vi "FPGAmain_5782_Dual_PID_v3.vi"() -> ()   [LabVIEW 2013]
uses:
  FPGA/DataMode.ctl
  FPGA/Input_5782/5782_states.ctl
  <vilib>/Platform/TimedLoop/XDataNode/timing_clust.ctl
  <vilib>/Platform/TimedLoop/XDataNode/nitl_modes.ctl
  <vilib>/Platform/TimedLoop/XDataNode/wakeup.ctl
  <vilib>/rvi/Emulation/niFpgaSctlEmulationGetInTimedLoop.vi
  <vilib>/rvi/Emulation/niFpgaEmulationReportErrorSimple.vi
  <vilib>/rvi/Emulation/niFpgaGetClockAttributes.vi
  <vilib>/rvi/eio/common/nirviEmuTemplateMethod_errors.vi
  <vilib>/rvi/Emulation/niFpgaCriticalErrorInLSC.vi
  <vilib>/rvi/DataTransferAndStorage/Register/Emulation/niFpgaRegisterEmulationFpgaImpl.vi
  <instcachedir>/0/niFpgaRegisterEmulationFpgaImpl_DCF4BC0110594B98B44A971D60CEEC4D.lvgen/niFpgaRegisterEmulationFpgaImpl_DCF4BC0110594B98B44A971D60CEEC4D_011.vi
  <vilib>/rvi/DataTransferAndStorage/Container/Common/niFpgaContainerGetUniqueNameForEmu.vi
  <instcachedir>/0/niFpgaRegisterEmulationFpgaImpl_DCF4BC0110594B98B44A971D60CEEC4D.lvgen/niFpgaRegisterEmulationFpgaImpl_DCF4BC0110594B98B44A971D60CEEC4D_012.vi
  <instcachedir>/0/niFpgaRegisterEmulationFpgaImpl_DCF4BC0110594B98B44A971D60CEEC4D.lvgen/niFpgaRegisterEmulationFpgaImpl_DCF4BC0110594B98B44A971D60CEEC4D_003.vi
  <instcachedir>/0/niFpgaRegisterEmulationFpgaImpl_DCF4BC0110594B98B44A971D60CEEC4D.lvgen/niFpgaRegisterEmulationFpgaImpl_DCF4BC0110594B98B44A971D60CEEC4D_007.vi
  <instcachedir>/0/niFpgaRegisterEmulationFpgaImpl_DCF4BC0110594B98B44A971D60CEEC4D.lvgen/niFpgaRegisterEmulationFpgaImpl_DCF4BC0110594B98B44A971D60CEEC4D_008.vi
  <instcachedir>/0/niFpgaRegisterEmulationFpgaImpl_DCF4BC0110594B98B44A971D60CEEC4D.lvgen/niFpgaRegisterEmulationFpgaImpl_DCF4BC0110594B98B44A971D60CEEC4D_021.vi
  <instcachedir>/0/niFpgaRegisterEmulationFpgaImpl_DCF4BC0110594B98B44A971D60CEEC4D.lvgen/niFpgaRegisterEmulationFpgaImpl_DCF4BC0110594B98B44A971D60CEEC4D_020.vi
  <instcachedir>/0/niFpgaRegisterEmulationFpgaImpl_DCF4BC0110594B98B44A971D60CEEC4D.lvgen/niFpgaRegisterEmulationFpgaImpl_DCF4BC0110594B98B44A971D60CEEC4D_009.vi
  <vilib>/rvi/FIFO/Fifo_Resource/nirvififoEmulationReadFpgaImpl.vi
  <vilib>/rvi/interface/RandomDataEmulation/nirviRandomDataMultiElementFPGAFIFO.vi
  <instcachedir>/0/nirviRandomDataMultiElementFPGAFIFO_F2B80EDE0D7944A08478D8D26097D4DB.lvgen/nirviRandomDataMultiElementFPGAFIFO_F2B80EDE0D7944A08478D8D26097D4DB_005.vi
  <vilib>/rvi/interface/RandomDataEmulation/niFpgaRandomDataHandleErrors.vi
  <instcachedir>/0/niFpgaRegisterEmulationFpgaImpl_DCF4BC0110594B98B44A971D60CEEC4D.lvgen/niFpgaRegisterEmulationFpgaImpl_DCF4BC0110594B98B44A971D60CEEC4D_013.vi
  <vilib>/rvi/interface/RandomDataEmulation/nirviRandomDataFPGAFIFO.vi
  <vilib>/rvi/FIFO/Fifo_Resource/nirvififoEmulationWriteFpgaImpl.vi
  <vilib>/Platform/TimedLoop/XDataNode/XDataNode.xnode
  <vilib>/eio/EIONode/EIONode.xnode
  <vilib>/rvi/DataTransferAndStorage/Container/XNode/niFpgaContainer.xnode
  <vilib>/rvi/DataTransferAndStorage/Register/Emulation/niFpgaRegisterEmulation.vi
  <vilib>/rvi/FIFO/Fifo_Resource/nirvififoEmulationRead.vi
  <vilib>/rvi/interface/RandomDataEmulation/nirviRandomDataFpgaMultiElementTemplate.vi
  <vilib>/rvi/interface/RandomDataEmulation/nirviRandomDataFpgaReadWriteTemplate.vi
  <vilib>/rvi/FIFO/Fifo_Resource/nirvififoEmulationWrite.vi
  <vilib>/Platform/TimedLoop/XDataNode/XDNodeRunTimeDep.lvlib
panel:
  in  "IO Module\\AO Data Sync":bool=TRUE
  in  "IO Module\\SPI Write Data":u16
  out "IO Module\\SPI Read Data":u8
  in  "IO Module\\SPI Read":bool
  in  "IO Module\\SPI Write":bool
  in  "IO Module\\SPI Address":u16
  in  "IO Module\\SPI Device":u8
  out "IO Module\\SPI Idle":bool
  in  "AM phase":fxp<+,64,64>
  in  "delay phase":fxp<+,64,64>
  in  "User Command Commit":bool
  in  "User Command":u8
  out "User Command Idle":bool
  out "User Command Status":u8
  in  "User Data 0":u8
  in  "User Data 1":u8
  out "PLL Locked":bool
  out "User Error":bool
  out "Configured?":bool
  in  "Continuous":bool
  in  "5782 record length":u16=4000 caption="Samples Per Trigger" min=1 step=1
  in  "Trigger Acquisition":bool
  out "IO Module\\Trigger Input":bool
  in  "Downsample":fxp<+,8,8>=1.0
  in  "new coeffs":bool
  in  "FIR coeffs":fxp<+/-,18,18>[](array[numeric])
  in  "CIC Gain":fxp<+/-,32,1>=0.00390625 format="%#_32g"
  in  "Acquisition running":bool
  in  "Phase output":fxp<+,64,64>[](array[numeric])=[0.0, 0.0, 0.0, 0.0, 0.0, 0.0, 0.0, 0.0]
  in  "Simulated phase 5782":fxp<+,64,64>[](array[numeric])=[0.0, 0.0]
  in  "Mode":T1
  in  "Phase 5782":fxp<+,64,64>[](array[numeric])=[0.0, 0.0]
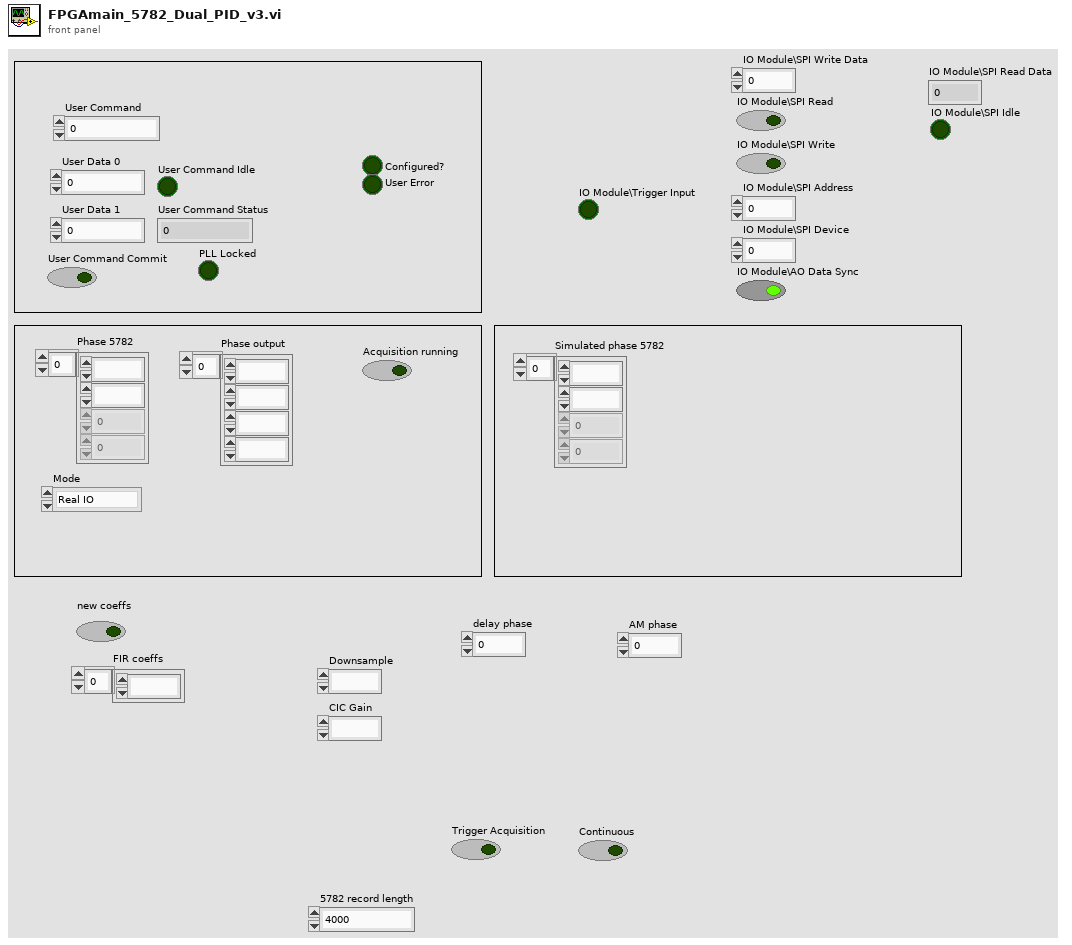
[diagram p1: front panel]
types:
  T1 = typedef "DataMode.ctl" = enum16{"Real IO", "Simulated"}
  T2 = typedef "5782_states.ctl" = enum8{"Wait for trigger", "Acquisition", "Send record length", "Quiet period"}
  T3 = typedef "XDNodeRunTimeDep.lvlib/timing_clust.ctl" = cluster{"Expected End [f-1]":u64, "Actual End [f-1]":u64, "Finished Late? [f-1]":bool, "Expected End [i-1]":u64, "Actual End [i-1]":u64, "Finished Late? [i-1]":bool, "Expected Start [i]":u64, "Actual Start [i]":u64, "Expected Start [f]":u64, "Actual Start [f]":u64, "Source Name":string, "Structure Name":string, "Period":i64, "Deadline":i64, "Offset":i64, "Start":i64, "Priority":i32, "Timeout":i32, "Mode":T4, "Wakeup Reason":T5, "Error":errorcluster, "Source Type":string, "Secondary Source Type":string, "Global End Time":u64, "Global Start Time":u64, "Frame Duration":u64, "Iteration Duration":u64, "Assigned CPU":i32, "I/O Scan Engine Mode":u32}
  T4 = typedef "XDNodeRunTimeDep.lvlib/nitl_modes.ctl" = enum32{"No Change", "Process missed periods, maintain original phase", "Discard missed periods, maintain original phase", "Process missed periods, ignore original phase", "Discard missed periods, ignore original phase"}
  T5 = typedef "XDNodeRunTimeDep.lvlib/wakeup.ctl" = enum32{"Normal", "Aborted", "Asynchronous wakeup", "Timing source error", "Timed loop error", "Timeout"}
  T6 = typedef "I16 array size 2.ctl" = i16[]
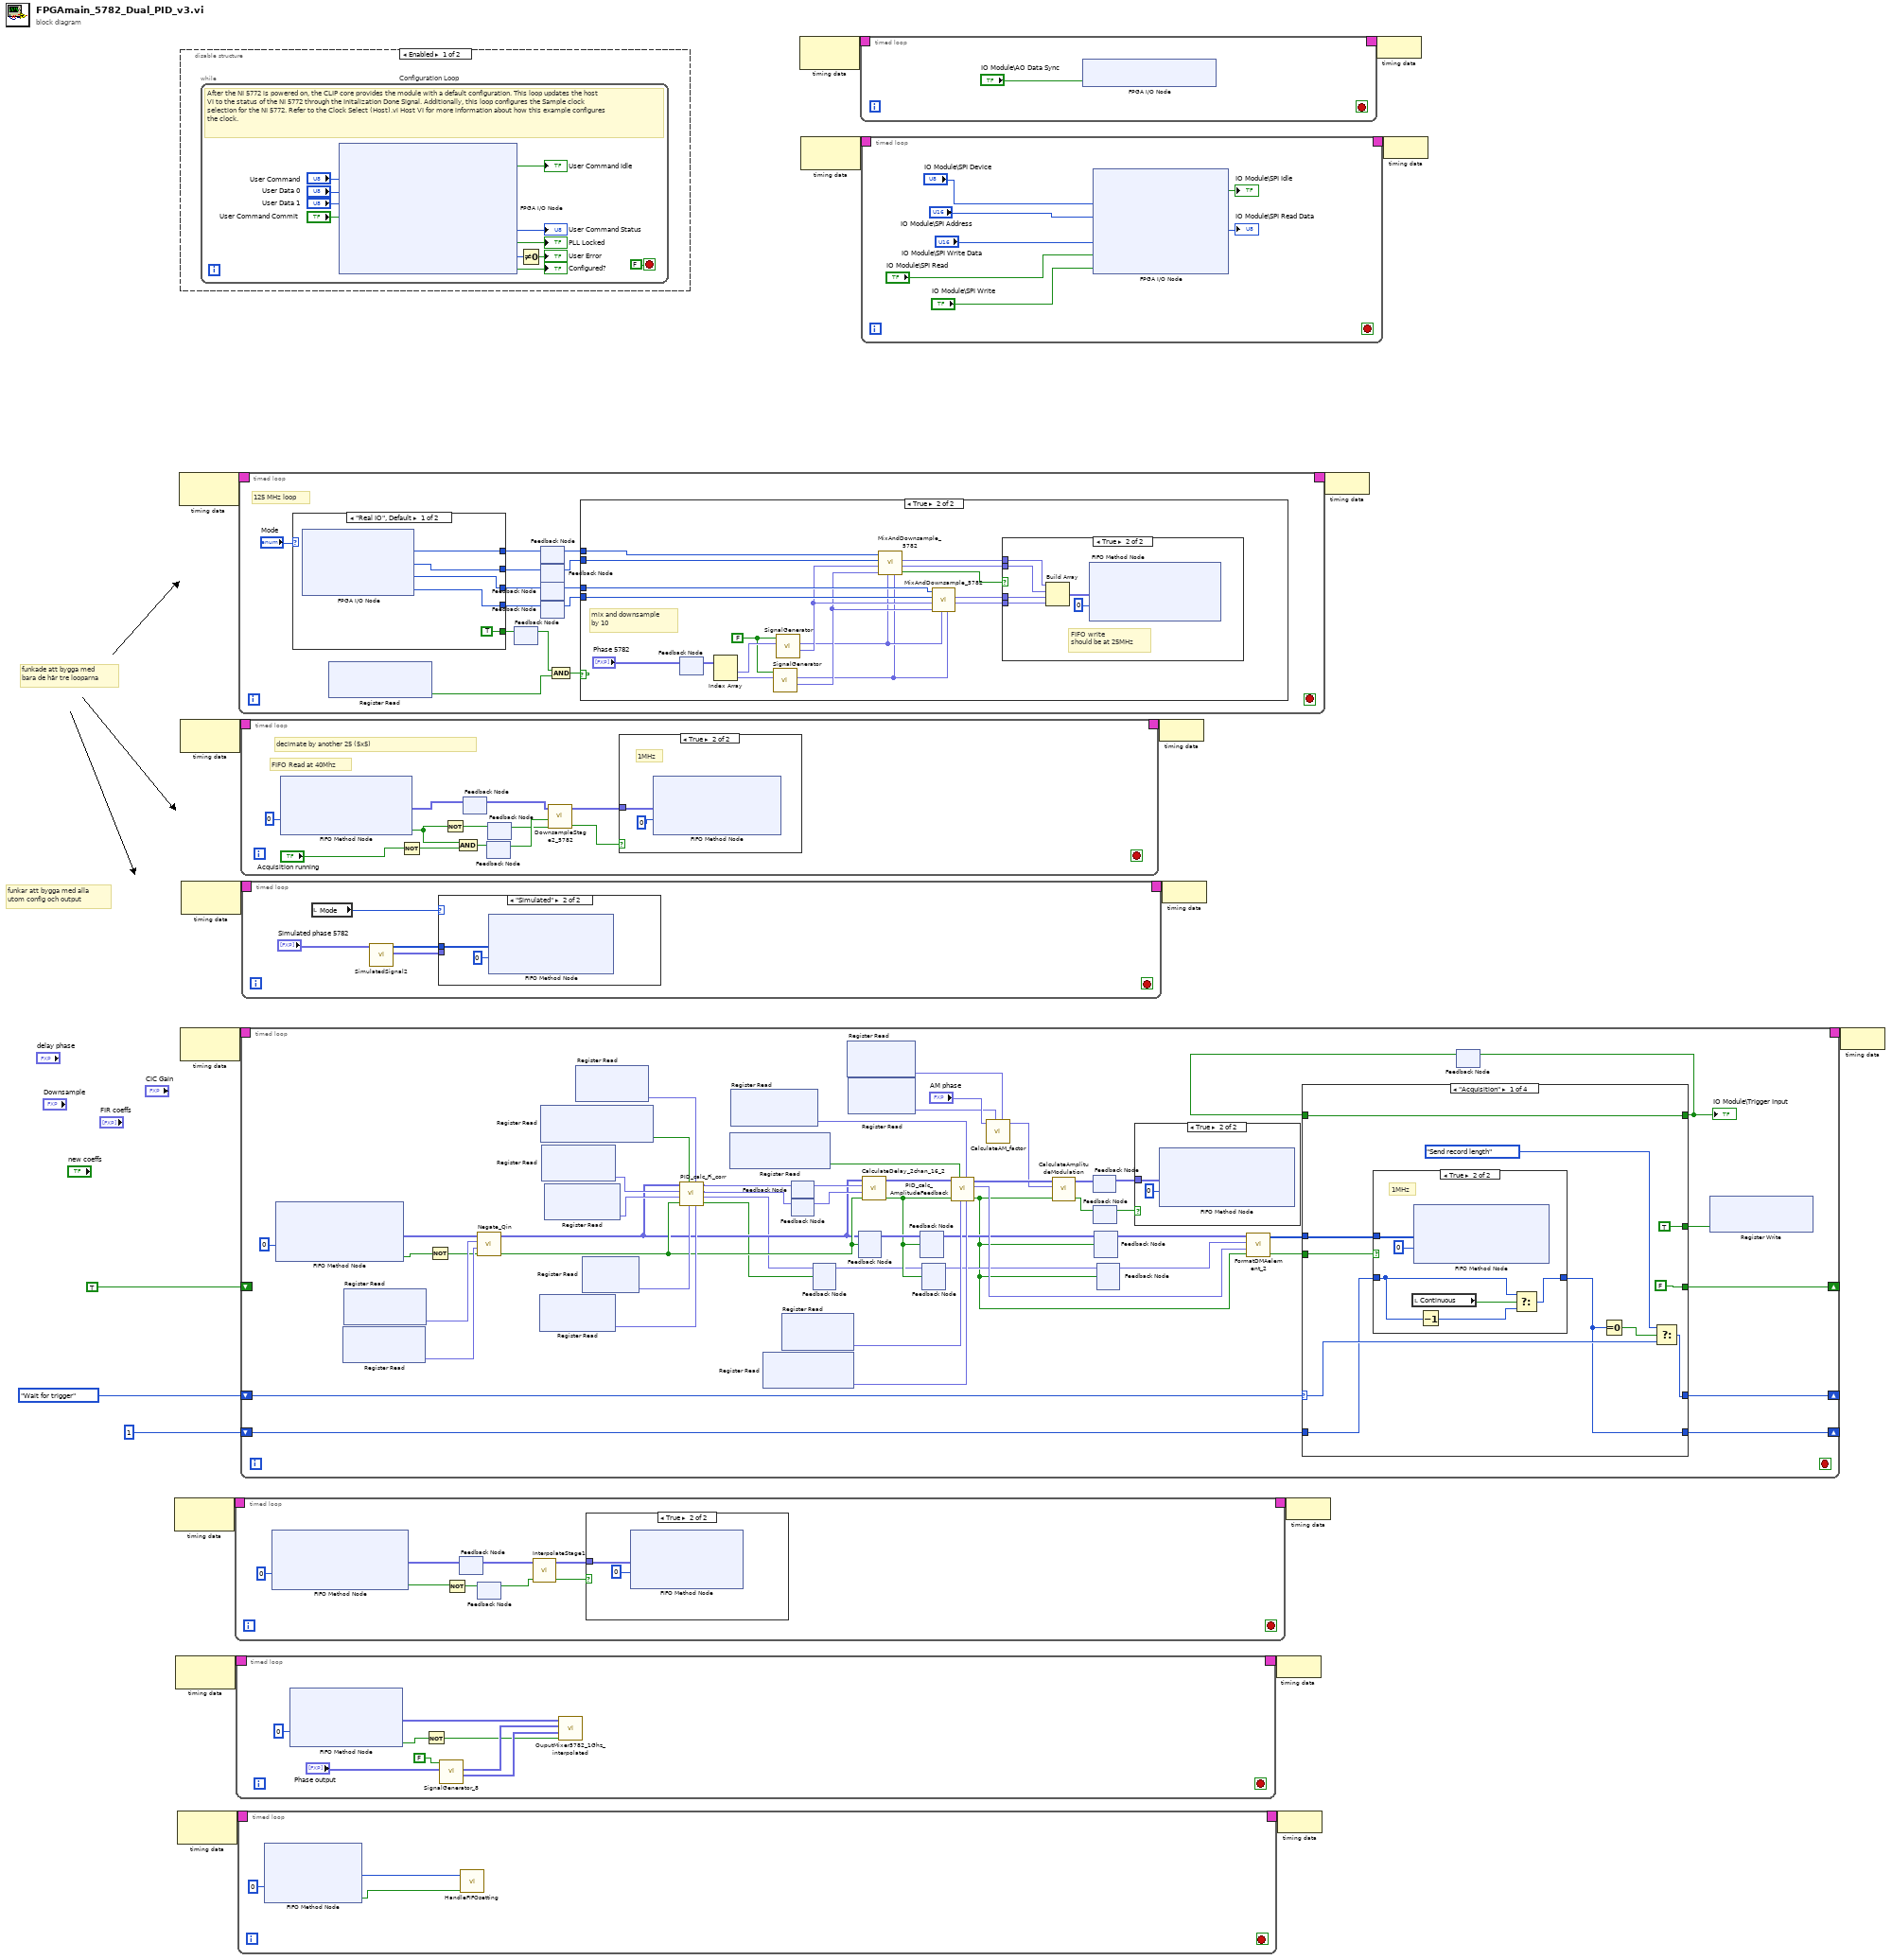
[diagram p0: block diagram]
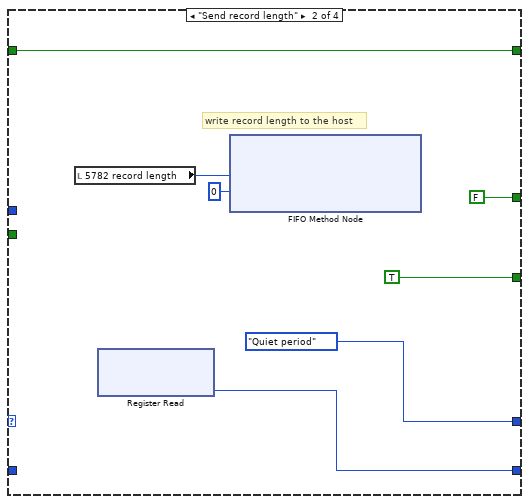
[diagram p5: hidden frame]
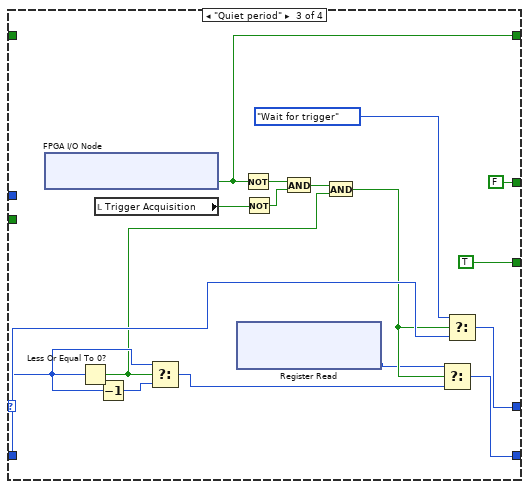
[diagram p6: hidden frame]
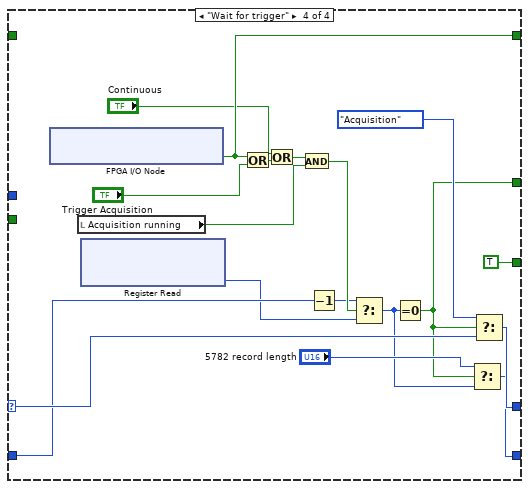
[diagram p7: hidden frame]
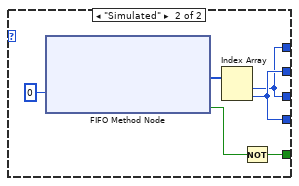
[diagram p11: hidden frame]
diagram:
  # "funkar att bygga med alla\nutom config och output"
  # "funkade att bygga med\nbara de här tre looparna"
  n1 = node-c288() -> (w2:T3)  [unwired: 1 in]
  n2 = node-c288() -> (w8:T3)  [unwired: 1 in]
  n3 = node-c288() -> (w10:T3)  [unwired: 1 in]
  n4 = node-c288() -> (w17:T3)  [unwired: 1 in]
  n5 = disable-structure shown="Enabled" {
    frame Enabled {
      n6 = while "Configuration Loop" {
        stop <- FALSE stop-if-true
        # "After the NI 5772 is powered on, the CLIP core provides the module with a default configuration. This loop updates the host VI to the status of the NI 5772 through the Initalization Done Signal. Additionally, this loop configures the Sample clock selection for the NI 5772. Refer to the Clock Select (Host).vi Host VI for more information about how this example configures the clock."
        n7 = xnode "FPGA I/O Node"("IO Module\\User Command"="User Command", "IO Module\\User Data 0"="User Data 0", "IO Module\\User Data 1"="User Data 1", "IO Module\\User Command Commit"="User Command Commit") -> ("IO Module\\User Command Idle"=→"User Command Idle":bool, "IO Module\\User Command Status"=→"User Command Status":u8, "IO Module\\PLL Locked"=→"PLL Locked":bool, "IO Module\\User Error"=w27:u8, "IO Module\\Initialization Done"=→"Configured?":bool)  [unwired: 9 in, 9 out]
        n8 = Not Equal To 0?(x=w27) -> (x != 0?=→"User Error":bool)
      }
    }
    frame Disabled {
    }
  }
  n9 = node-c288() -> (w21:T3)  [unwired: 1 in]
  n10 = node-c288() -> (w15:T3)  [unwired: 1 in]
  n11 = node-c288() -> (w19:T3)  [unwired: 1 in]
  n12 = timed-loop {
    timing: w2 -> [_]
    timing-out: [_] -> w1
    stop <- _ stop-if-true
    n13 = xnode ("FIFO Method Node")("Timeout"=0) -> ("Element"=w34:fxp<+/-,16,14>[], "Timed Out?"=w39:bool)  [unwired: 1 in, 1 out]
    n14 = Not(x=w39) -> (.not. x?=w36:bool)
    n15 = feedback #1() -> (w33:fxp<+/-,16,14>[])  [unwired: 1 in]
    n16 = feedback-in #1(w34) -> ()
    n17 = feedback #2() -> (w35:bool)  [unwired: 1 in]
    n18 = feedback-in #2(w36) -> ()
    n19 = call "InterpolateStage1.vi"("valid in"=w35, "Data in"=w33) -> ("valid out"=w38:bool, "Data out"=w37:fxp<+/-,16,14>[])  [unwired: 8 in]
    n20 = case shown="True" w38 {
      tunnel: w37 -> [_ w42]
      frame False {
      }
      frame True {
        n21 = xnode ("FIFO Method Node")("Element"=w42, "Timeout"=0) -> ()  [unwired: 1 in, 2 out]
      }
    }
  }
  n22 = timed-loop {
    timing: w8 -> [_]
    timing-out: [_] -> w7
    stop <- _ stop-if-true
    n23 = xnode ("FIFO Method Node")("Timeout"=0) -> ("Element"=w46:fxp<+/-,16,14>[], "Timed Out?"=w51:bool)  [unwired: 1 in, 1 out]
    n24 = Not(x=w51) -> (.not. x?=w45:bool)
    n25 = call "SignalGenerator_8.vi"("Phase"="Phase output", "reset"=FALSE) -> ("Sine out"=w47:fxp<+/-,16,0>[], "Cosine out"=w48:fxp<+/-,16,0>[])  [unwired: 8 in]
    n26 = call "OuputMixer5782_1Ghz_interpolated.vi"("input valid"=w45, "Sine in"=w47, "Cosine in"=w48, "Data"=w46) -> ()  [unwired: 7 in, 1 out]
  }
  n27 = timed-loop {
    timing: w10 -> [_]
    timing-out: [_] -> w9
    stop <- _ stop-if-true
    n28 = xnode ("FIFO Method Node")("Timeout"=0) -> ("Element"=w56:u64, "Timed Out?"=w55:bool)  [unwired: 1 in, 1 out]
    n29 = call "HandleFIFOsetting.vi"("timed out"=w55, "Value"=w56) -> ()  [unwired: 10 in]
  }
  n30 = timed-loop {
    timing: w17 -> [_]
    timing-out: [_] -> w16
    stop <- _ stop-if-true
    # "125 MHz loop"
    n31 = case shown="\"Real IO\", Default" "Mode" {
      tunnel: [w101 w104] -> w70
      tunnel: [w100 w105] -> w68
      tunnel: [w99 w104] -> w66
      tunnel: [w98 w105] -> w63
      tunnel: [TRUE w102] -> w62
      frame "Real IO", Default {
        n32 = xnode "FPGA I/O Node"() -> ("IO Module\\AI 0 N-1"=w101:i16, "IO Module\\AI 0 N"=w100:i16, "IO Module\\AI 1 N-1"=w99:i16, "IO Module\\AI 1 N"=w98:i16)  [unwired: 4 in, 4 out]
      }
      frame "Simulated" {
        n33 = xnode ("FIFO Method Node")("Timeout"=0) -> ("Element"=w106:i16[], "Timed Out?"=w103:bool)  [unwired: 1 in, 1 out]
        n34 = Index Array(array=w106) -> (element #1=w104:i16, element #2=w105:i16)  [unwired: 2 in]
        n35 = Not(x=w103) -> (.not. x?=w102:bool)
      }
    }
    n36 = xnode ("Register Read")() -> ("Data"=w60:bool)  [unwired: 1 in, 1 out]
    n37 = feedback #3() -> (w61:bool)  [unwired: 1 in]
    n38 = feedback-in #3(w62) -> ()
    n39 = feedback #4() -> (w69:i16)  [unwired: 1 in]
    n40 = feedback-in #4(w70) -> ()
    n41 = feedback #5() -> (w67:i16)  [unwired: 1 in]
    n42 = feedback-in #5(w68) -> ()
    n43 = feedback #6() -> (w65:i16)  [unwired: 1 in]
    n44 = feedback-in #6(w66) -> ()
    n45 = feedback #7() -> (w64:i16)  [unwired: 1 in]
    n46 = feedback-in #7(w63) -> ()
    n47 = And(x=w61, y=w60) -> (x .and. y?=w71:bool)
    n48 = case shown="True" w71 {
      tunnel: w69 -> [_ w80]
      tunnel: w67 -> [_ w79]
      tunnel: w65 -> [_ w78]
      tunnel: w64 -> [_ w77]
      frame False {
      }
      frame True {
        w81 = FALSE
        # "mix and downsample\nby 10"
        n49 = feedback #8() -> (w84:fxp<+,64,64>[])  [unwired: 1 in]
        n50 = feedback-in #8("Phase 5782") -> ()
        n51 = Index Array(array=w84) -> (element #1=w83:fxp<+,64,64>, element #2=w85:fxp<+,64,64>)  [unwired: 2 in]
        n52 = call "SignalGenerator.vi"("phase"=w85, "Reset"=w81) -> ("Cos"=w75:fxp<+/-,16,0>, "Sin"=w73:fxp<+/-,16,0>)  [unwired: 7 in, 1 out]
        n53 = call "SignalGenerator.vi"("phase"=w83, "Reset"=w81) -> ("Cos"=w76:fxp<+/-,16,0>, "Sin"=w74:fxp<+/-,16,0>)  [unwired: 7 in, 1 out]
        n54 = call "MixAndDownsample_5782.vi"("sin1"=w73, "sin0"=w74, "cos1"=w75, "cos0"=w76, "signal 1"=w79, "signal 0"=w80) -> ("data valid"=w88:bool, "Q out"=w89:fxp<+/-,16,14>, "I out"=w90:fxp<+/-,16,14>)  [unwired: 3 in]
        n55 = call "MixAndDownsample_5782.vi"("sin1"=w73, "sin0"=w74, "cos1"=w75, "cos0"=w76, "signal 1"=w77, "signal 0"=w78) -> ("Q out"=w86:fxp<+/-,16,14>, "I out"=w87:fxp<+/-,16,14>)  [unwired: 3 in, 1 out]
        n56 = case shown="True" w88 {
          tunnel: w89 -> [_ w96]
          tunnel: w90 -> [_ w93]
          tunnel: w87 -> [_ w92]
          tunnel: w86 -> [_ w91]
          frame False {
          }
          frame True {
            # "FIFO write\nshould be at 25MHz"
            n57 = Build Array(w93, w96, w92, w91) -> (w95:fxp<+/-,16,14>[])
            n58 = xnode ("FIFO Method Node")("Element"=w95, "Timeout"=0) -> ()  [unwired: 1 in, 2 out]
          }
        }
      }
    }
  }
  n59 = timed-loop {
    timing: w21 -> [_]
    timing-out: [_] -> w20
    stop <- _ stop-if-true
    # "FIFO Read at 40Mhz"
    # "decimate by another 25 (5x5)"
    n60 = xnode ("FIFO Method Node")("Timeout"=0) -> ("Element"=w115:fxp<+/-,16,14>[], "Timed Out?"=w117:bool)  [unwired: 1 in, 1 out]
    n61 = Not(x="Acquisition running") -> (.not. x?=w118:bool)
    n62 = Not(x=w117) -> (.not. x?=w111:bool)
    n63 = And(x=w117, y=w118) -> (x .and. y?=w113:bool)
    n64 = feedback #9() -> (w114:fxp<+/-,16,14>[])  [unwired: 1 in]
    n65 = feedback-in #9(w115) -> ()
    n66 = feedback #10() -> (w112:bool)  [unwired: 1 in]
    n67 = feedback-in #10(w113) -> ()
    n68 = feedback #11() -> (w110:bool)  [unwired: 1 in]
    n69 = feedback-in #11(w111) -> ()
    n70 = call "DownsampleStage2_5782.vi"("valid in"=w110, "reset"=w112, "Data in"=w114) -> ("valid out"=w119:bool, "data out"=w120:fxp<+/-,16,14>[])  [unwired: 7 in]
    n71 = case shown="True" w119 {
      tunnel: w120 -> [_ w122]
      frame False {
      }
      frame True {
        # "1MHz"
        n72 = xnode ("FIFO Method Node")("Element"=w122, "Timeout"=0) -> ()  [unwired: 1 in, 2 out]
      }
    }
  }
  n73 = timed-loop {
    timing: w15 -> [_]
    timing-out: [_] -> w14
    shift-right: [w176] -> _
    shift-left: 5782_states."Wait for trigger" ("5782 states") -> [w178]
    shift-right: [w175] -> _
    shift-left: u16 1 ("trigger samples") -> [w177]
    shift-right: [w170] -> _
    shift-left: TRUE -> [_]
    stop <- _ stop-if-true
    n74 = xnode ("FIFO Method Node")("Timeout"=0) -> ("Element"=w156:fxp<+/-,16,14>[], "Timed Out?"=w173:bool)  [unwired: 1 in, 1 out]
    n75 = xnode ("Register Read")() -> ("Data"=w163:fxp<+/-,16,14>)  [unwired: 1 in, 1 out]
    n76 = xnode ("Register Read")() -> ("Data"=w164:fxp<+/-,16,14>)  [unwired: 1 in, 1 out]
    n77 = Not(x=w173) -> (.not. x?=w157:bool)
    n78 = call "Negate_Qin.vi"("valid in"=w157, "DC offset chan 1"=w163, "DC offset chan 0"=w164, "Data in"=w156) -> ("valid out"=w143:bool, "Data out"=w142:fxp<+/-,16,14>[])  [unwired: 6 in]
    n79 = xnode ("Register Read")() -> ("Data"=w150:fxp<+/-,32,4>)  [unwired: 1 in, 1 out]
    n80 = xnode ("Register Read")() -> ("Data"=w147:bool)  [unwired: 1 in, 1 out]
    n81 = xnode ("Register Read")() -> ("Data"=w148:fxp<+/-,32,4>)  [unwired: 1 in, 1 out]
    n82 = xnode ("Register Read")() -> ("Data"=w149:fxp<+/-,32,4>)  [unwired: 1 in, 1 out]
    n83 = xnode ("Register Read")() -> ("Data"=w146:fxp<+/-,32,4>)  [unwired: 1 in, 1 out]
    n84 = xnode ("Register Read")() -> ("Data"=w151:fxp<+/-,32,4>)  [unwired: 1 in, 1 out]
    n85 = call "PID_calc_Fi_corr.vi"("Kd/Tau"=w150, "Ki*Tau"=w146, "Kp"=w151, "Enabled"=w147, "input valid"=w143, "Fi_delta"=w149, "Fi_start"=w148, "Data in"=w142) -> ("output valid"=w140:bool, "c out"=w141:fxp<+/-,32,4>, "cos_fi_korr"=w144:fxp<+/-,16,2>, "sin fi_korr"=w145:fxp<+/-,16,2>)
    n86 = xnode ("Register Read")() -> ("Data"=w161:bool)  [unwired: 1 in, 1 out]
    n87 = xnode ("Register Read")() -> ("Data"=w158:fxp<+/-,32,6>)  [unwired: 1 in, 1 out]
    n88 = xnode ("Register Read")() -> ("Data"=w159:fxp<+/-,32,6>)  [unwired: 1 in, 1 out]
    n89 = xnode ("Register Read")() -> ("Data"=w160:fxp<+/-,32,6>)  [unwired: 1 in, 1 out]
    n90 = feedback-in #12(w145) -> ()
    n91 = feedback #12() -> (w166:fxp<+/-,16,2>)  [unwired: 1 in]
    n92 = feedback #13() -> (w165:fxp<+/-,16,2>)  [unwired: 1 in]
    n93 = feedback-in #13(w144) -> ()
    n94 = feedback #14() -> (w135:fxp<+/-,32,4>)  [unwired: 1 in]
    n95 = feedback-in #14(w141, w140) -> ()
    n96 = xnode ("Register Read")() -> ("Data"=w128:fxp<+/-,16,2>)  [unwired: 1 in, 1 out]
    n97 = xnode ("Register Read")() -> ("Data"=w129:fxp<+/-,16,2>)  [unwired: 1 in, 1 out]
    n98 = feedback #15() -> (w138:fxp<+/-,16,14>[])  [unwired: 1 in]
    n99 = feedback-in #15(w142, w143) -> ()
    n100 = call "CalculateDelay_2chan_16_2.vi"("input valid"=w143, "cos_fi"=w165, "sin fi"=w166, "Data in"=w142) -> ("output valid"=w136:bool, "Data out"=w162:fxp<+/-,16,14>[])  [unwired: 6 in]
    n101 = feedback #16() -> (w137:fxp<+/-,16,14>[])  [unwired: 1 in]
    n102 = feedback-in #16(w138, w136) -> ()
    n103 = feedback #17() -> (w134:fxp<+/-,32,4>)  [unwired: 1 in]
    n104 = feedback-in #17(w135, w136) -> ()
    n105 = call "PID_calc_AmplitudeFeedback.vi"("Kd/Tau"=w159, "Ki*Tau"=w158, "Kp"=w160, "Enabled"=w161, "input valid"=w136, "Data in"=w162) -> ("output valid"=w131:bool, "c(t)"=w152:fxp<+/-,32,21>, "data out"=w133:fxp<+/-,16,14>[])  [unwired: 2 in, 1 out]
    n106 = call "CalculateAM_factor.vi"("b_am"=w128, "a_am"=w129, "AM phase"="AM phase") -> ("AM_factor"=w127:fxp<+/-,16,2>)  [unwired: 7 in, 1 out]
    n107 = call "CalculateAmplitudeModulation.vi"("input valid"=w131, "AM_factor"=w127, "Data in"=w133) -> ("output valid"=w126:bool, "Data out"=w132:fxp<+/-,16,14>[])  [unwired: 7 in]
    n108 = feedback #18() -> (w155:fxp<+/-,16,14>[])  [unwired: 1 in]
    n109 = feedback-in #18(w132) -> ()
    n110 = feedback #19() -> (w154:bool)  [unwired: 1 in]
    n111 = feedback-in #19(w126) -> ()
    n112 = feedback #20() -> (w153:fxp<+/-,16,14>[])  [unwired: 1 in]
    n113 = feedback-in #20(w137, w131) -> ()
    n114 = feedback #21() -> (w139:fxp<+/-,32,4>)  [unwired: 1 in]
    n115 = feedback-in #21(w134, w131) -> ()
    n116 = case shown="True" w154 {
      tunnel: w155 -> [_ w179]
      frame False {
      }
      frame True {
        n117 = xnode ("FIFO Method Node")("Element"=w179, "Timeout"=0) -> ()  [unwired: 1 in, 2 out]
      }
    }
    n118 = call "FormatDMAelement_2.vi"("valid in"=w131, "c(t) - AM"=w152, "c(t) - Phase"=w139, "Data in"=w153) -> ("valid out"=w171:bool, "Element"=w172:u64[])  [unwired: 6 in]
    n119 = feedback #22() -> (w168:bool)  [unwired: 1 in]
    n120 = case shown="\"Acquisition\"" w178 {
      selector: w178 -> [w191 _ w221 w240]
      tunnel: w177 -> [w187 _ w209 w227]
      tunnel: [w190 5782_states."Quiet period" ("5782 states") w220 w239] -> w176
      tunnel: [w184 w199 w222 w238] -> w175
      tunnel: w172 -> [w185 _ _ _]
      tunnel: w171 -> [w186 _ _ _]
      tunnel: [FALSE TRUE TRUE TRUE] -> w170
      tunnel: [TRUE FALSE ("5782 triggered") FALSE ("5782 triggered") w231] -> w169
      tunnel: [w183 w200 w211 w230] -> w167
      tunnel: w168 -> [w183 w200 _ _]
      frame "Acquisition" {
        n121 = case shown="True" w186 {
          tunnel: w185 -> [_ w198]
          tunnel: [w192 w195] -> w184
          tunnel: w187 -> [w192 w193]
          frame False {
          }
          frame True {
            # "1MHz"
            n122 = local read "Continuous"() -> (w196:bool)
            n123 = xnode ("FIFO Method Node")("Element"=w198, "Timeout"=0) -> ()  [unwired: 1 in, 2 out]
            n124 = Decrement(x=w193) -> (x-1=w194:u16)
            n125 = Select(t=w193, s=w196, f=w194) -> (s? t:f=w195:u16)
          }
        }
        n126 = Equal To 0?(x=w184) -> (x = 0?=w188:bool)
        n127 = Select(t=5782_states."Send record length" ("5782 states"), s=w188, f=w191) -> (s? t:f=w190:T2)
      }
      frame "Send record length" {
        # "write record length to the host"
        n128 = local read "5782 record length"() -> (w202:u16)
        n129 = xnode ("Register Read")() -> ("Data"=w199:u16)  [unwired: 1 in, 1 out]
        n130 = xnode ("FIFO Method Node")("Element"=w202, "Timeout"=0) -> ()  [unwired: 1 in, 2 out]
      }
      frame "Quiet period" {
        n131 = xnode "FPGA I/O Node"() -> ("IO Module\\Trigger Input"=w211:bool)  [unwired: 1 in, 1 out]
        n132 = Less Or Equal To 0?(x=w209) -> (x <= 0?=w208:bool)
        n133 = local read "Trigger Acquisition"() -> (w217:bool)
        n134 = Decrement(x=w209) -> (x-1=w210:u16)
        n135 = Select(t=w209, s=w208, f=w210) -> (s? t:f=w207:u16)
        n136 = xnode ("Register Read")() -> ("Data"=w206:u16)  [unwired: 1 in, 1 out]
        n137 = Not(x=w211) -> (.not. x?=w216:bool)
        n138 = Not(x=w217) -> (.not. x?=w215:bool)
        n139 = And(x=w216, y=w215) -> (x .and. y?=w214:bool)
        n140 = And(x=w214, y=w208) -> (x .and. y?=w219:bool)
        n141 = Select(t=w206, s=w219, f=w207) -> (s? t:f=w222:u16)
        n142 = Select(t=5782_states."Wait for trigger" ("5782 states"), s=w219, f=w221) -> (s? t:f=w220:T2)
      }
      frame "Wait for trigger" {
        n143 = xnode "FPGA I/O Node"() -> ("IO Module\\Trigger Input"=w230:bool)  [unwired: 1 in, 1 out]
        n144 = local read "Acquisition running"() -> (w232:bool)
        n145 = xnode ("Register Read")() -> ("Data"=w223:u16)  [unwired: 1 in, 1 out]
        n146 = Or(x=w230, y="Trigger Acquisition") -> (x .or. y?=w226:bool)
        n147 = Or(x="Continuous", y=w226) -> (x .or. y?=w224:bool)
        n148 = And(x=w224, y=w232) -> (x .and. y?=w233:bool)
        n149 = Decrement(x=w227) -> (x-1=w228:u16)
        n150 = Select(t=w228, s=w233, f=w223) -> (s? t:f=w229:u16)
        n151 = Equal To 0?(x=w229) -> (x = 0?=w231:bool)
        n152 = Select(t="5782 record length", s=w231, f=w229) -> (s? t:f=w238:u16)
        n153 = Select(t=5782_states."Acquisition" ("5782 states"), s=w231, f=w240) -> (s? t:f=w239:T2)
      }
    }
    "IO Module\\Trigger Input" <- w167
    n154 = feedback-in #22(w167) -> ()
    n155 = xnode ("Register Write")("Data"=w169) -> ()  [unwired: 1 in, 1 out]
  }
  n156 = timed-loop {
    timing: w19 -> [_]
    timing-out: [_] -> w18
    stop <- _ stop-if-true
    n157 = local read "Mode"() -> (w246:T1)
    n158 = call "SimulatedSignal2.vi"("Phase"="Simulated phase 5782") -> ("dummy do not use"=w243:fxp<+/-,16,0>[], "output"=w245:T6)  [unwired: 9 in]
    n159 = case shown="\"Simulated\"" w246 {
      tunnel: w245 -> [_ w247]
      tunnel: w243 -> [_ _]
      frame "Real IO", Default {
      }
      frame "Simulated" {
        n160 = xnode ("FIFO Method Node")("Element"=w247, "Timeout"=0) -> ()  [unwired: 1 in, 2 out]
      }
    }
  }
  n161 = node-c288() -> (w4:T3)  [unwired: 1 in]
  n162 = node-c288() -> (w6:T3)  [unwired: 1 in]
  n163 = timed-loop {
    timing: w4 -> [_]
    timing-out: [_] -> w3
    stop <- _ stop-if-true
    n164 = xnode "FPGA I/O Node"("IO Module\\AO Data Sync"="IO Module\\AO Data Sync") -> ()  [unwired: 1 in, 1 out]
  }
  n165 = timed-loop {
    timing: w6 -> [_]
    timing-out: [_] -> w5
    stop <- _ stop-if-true
    n166 = xnode "FPGA I/O Node"("IO Module\\SPI Device"="IO Module\\SPI Device", "IO Module\\SPI Address"="IO Module\\SPI Address", "IO Module\\SPI Write Data"="IO Module\\SPI Write Data", "IO Module\\SPI Read"="IO Module\\SPI Read", "IO Module\\SPI Write"="IO Module\\SPI Write") -> ("IO Module\\SPI Idle"=→"IO Module\\SPI Idle":bool, "IO Module\\SPI Read Data"=→"IO Module\\SPI Read Data":u8)  [unwired: 7 in, 7 out]
  }
  n167 = node-c288(w20) -> ()
  n168 = node-c288(w18) -> ()
  n169 = node-c288(w7) -> ()
  n170 = node-c288(w9) -> ()
  n171 = node-c288(w1) -> ()
  n172 = node-c288(w16) -> ()
  n173 = node-c288(w3) -> ()
  n174 = node-c288(w5) -> ()
  n175 = node-c288(w14) -> ()
